vi "SquareWaveComp.vi"(6 "Amp":dbl=10.0 format="%#_13g", 8 "Offset":dbl=10.0 format="%#_13g", 9 "sampling info":cluster{"Fs":dbl, "#s":dbl}={"Fs"=100.0, "#s"=1600.0}, 10 "frequency":dbl=0.0625 format="%#_13g", 11 "Components":i32=3) -> (3 "Decomposed":dbl[](array[numeric]))   [LabVIEW 2016]
uses:
  <vilib>/measure/NI_MABase.lvlib
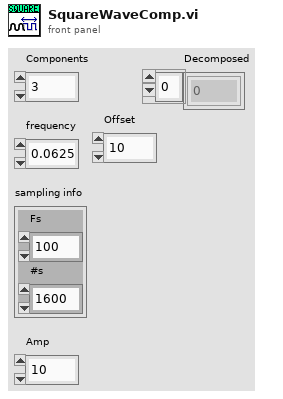
[diagram p1: front panel]
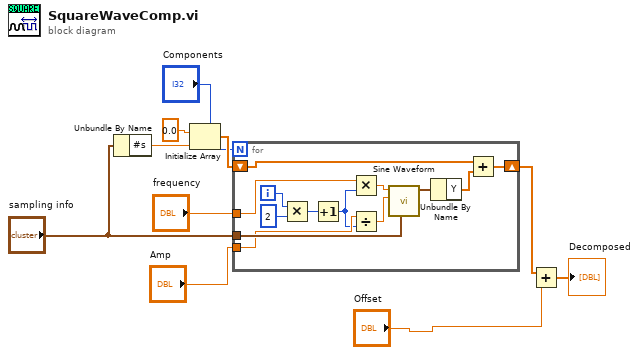
[diagram p0: block diagram]
diagram:
  n1 = Unbundle By Name("sampling info") -> ("#s"=w10:dbl)
  n2 = Initialize Array(0.0 ("element"), w10) -> (w7:dbl[])
  n3 = for {
    N: "Components" -> [_]
    tunnel: "sampling info" -> [w23]
    shift-right: [w15] -> w4
    shift-left: w7 -> [w16]
    tunnel: "Amp" -> [w22]
    tunnel: "frequency" -> [w20]
    i -> [w14]
    n4 = Multiply(x=w14, y=2) -> (x*y=w12:i32)
    n5 = Increment(x=w12) -> (x+1=w11:i32)
    n6 = Multiply(x=w20, y=w11) -> (x*y=w19:dbl)
    n7 = Divide(x=w22, y=w11) -> (x/y=w21:dbl)
    n8 = call <vilib>:"Sine Waveform.vi"("sampling info"=w23, "amplitude"=w21, "frequency"=w19) -> ("signal out"=w18:waveform(dbl))  [unwired: 7 in, 1 out]
    n9 = Unbundle By Name(w18) -> ("Y"=w17:dbl[])
    n10 = Add(x=w16, y=w17) -> (x+y=w15:dbl[])
  }
  n11 = Add(x=w4, y="Offset") -> (x+y=→"Decomposed":dbl[])
